vi "MFC_SV_Combined.vi"(9 "SV Array 1Hz":bool[](array[boolean]), 10 "SV Array 5Hz":bool[](array[boolean])) -> (2 "SV Full MFC":bool[](array[boolean]))   [LabVIEW 2014]
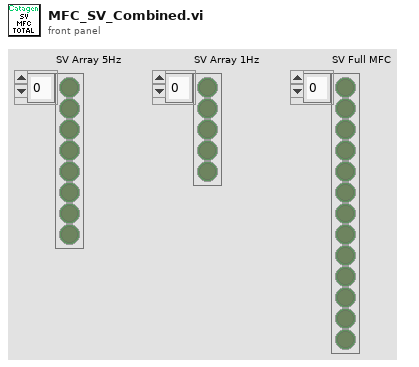
[diagram p1: front panel]
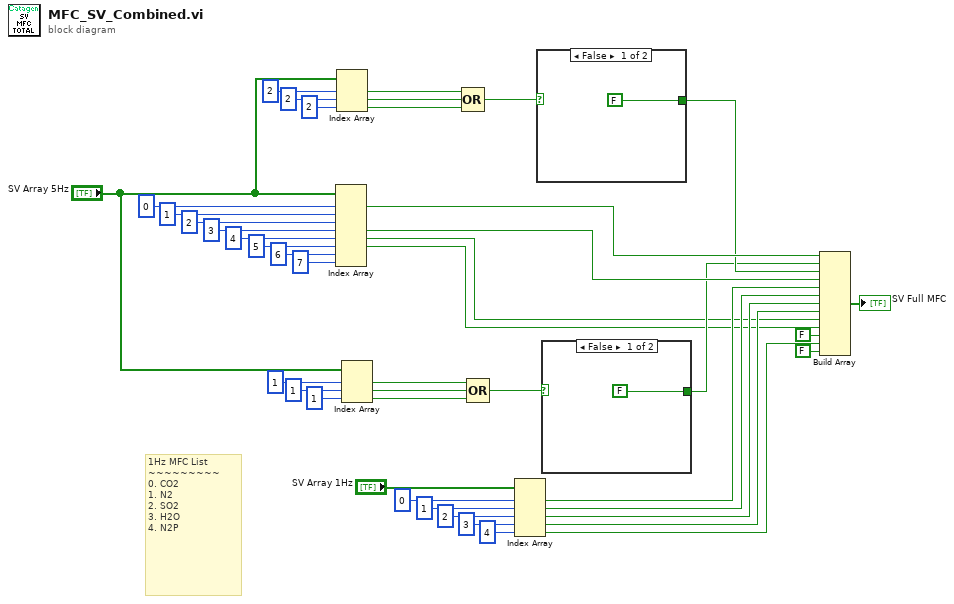
[diagram p0: block diagram]
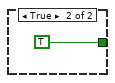
[diagram p2: hidden frame]
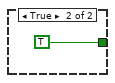
[diagram p3: hidden frame]
diagram:
  # "1Hz MFC List\n~~~~~~~~~\n0. CO2\n1. N2\n2. SO2\n3. H2O\n4. N2P"
  n1 = Index Array(array="SV Array 5Hz", index #1=0 ("index"), index #2=1 ("index"), index #3=2 ("index"), index #4=3 ("index"), index #5=4 ("index"), index #6=5 ("index"), index #7=6 ("index"), index #8=7 ("index")) -> (element #1=w32:bool, element #4=w31:bool, element #5=w1:bool, element #6=w2:bool)  [unwired: 4 out]
  n2 = Index Array(array="SV Array 5Hz", index #1=2 ("index"), index #2=2 ("index"), index #3=2 ("index")) -> (element #1=w17:bool, element #2=w16:bool, element #3=w15:bool)
  n3 = Index Array(array="SV Array 5Hz", index #1=1 ("index"), index #2=1 ("index"), index #3=1 ("index")) -> (element #1=w8:bool, element #2=w9:bool, element #3=w10:bool)
  n4 = Compound Arithmetic op=OR(w17, w16, w15) -> (w14:bool)
  n5 = Compound Arithmetic op=OR(w8, w9, w10) -> (w11:bool)
  n6 = Index Array(array="SV Array 1Hz", index #1=0 ("index"), index #2=1 ("index"), index #3=2 ("index"), index #4=3 ("index"), index #5=4 ("index")) -> (element #1=w37:bool, element #2=w36:bool, element #3=w35:bool, element #4=w34:bool, element #5=w33:bool)
  n7 = case shown="False" w14 {
    tunnel: [FALSE ("element") TRUE ("element")] -> w13
    frame False {
    }
    frame True {
    }
  }
  n8 = case shown="False" w11 {
    tunnel: [FALSE ("element") TRUE ("element")] -> w3
    frame False {
    }
    frame True {
    }
  }
  n9 = Build Array(w32, w3, w13, w31, w37, w36, w35, w34, w1, w2, FALSE ("element"), w33, FALSE ("element")) -> (→"SV Full MFC":bool[])
